vi "SubpanelClosedHandler.vi"(8 "error in (no error)":errorcluster, 9 "UI State":T1=enum."Embedded", 10 "EmbeddedSMO":refnum<class "SMO.UI.Embedded.lvclass">, 11 "SMO.UI.MAUI in":refnum<class "SMO.UI.MAUI.lvclass">) -> (0 "error out":errorcluster, 3 "SMO.UI.MAUI out":refnum<class "SMO.UI.MAUI.lvclass">)   [LabVIEW 2016, in "SMO.UI.MAUI.lvclass"]
uses:
  SMO.UI.MAUI.lvclass
  <vilib>/Levylab/SMO.UI.Embedded/SMO.UI.Embedded.lvclass
  C:/Program Files (x86)/National Instruments/LabVIEW 2016/vi.lib/JKI/JKI SMO/SMO/SMO.lvclass
  <vilib>/Levylab/SMO.UI.Embedded/Typedefs/UI State.ctl
  SMO.UI.MAUI.lvclass/SMO.UI.MAUI.ctl
  <vilib>/JKI/JKI SMO/SMO/SMO.lvclass
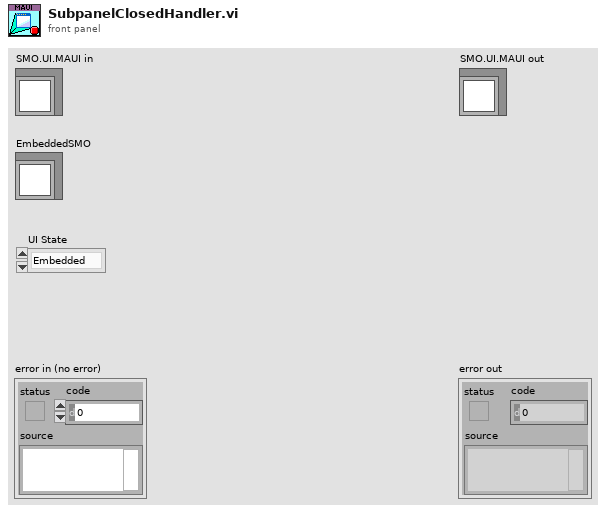
[diagram p1: front panel]
types:
  T1 = typedef "SMO.UI.Embedded.lvclass/UI State.ctl" = enum16{"unknown", "Opened", "Embedded", "Closed"}
  T2 = typedef "SMO.UI.MAUI.lvclass/PanelData.ctl" = cluster{"SubPanel":refnum<vi>, "Ring":refnum<vi>, "Active":i32}
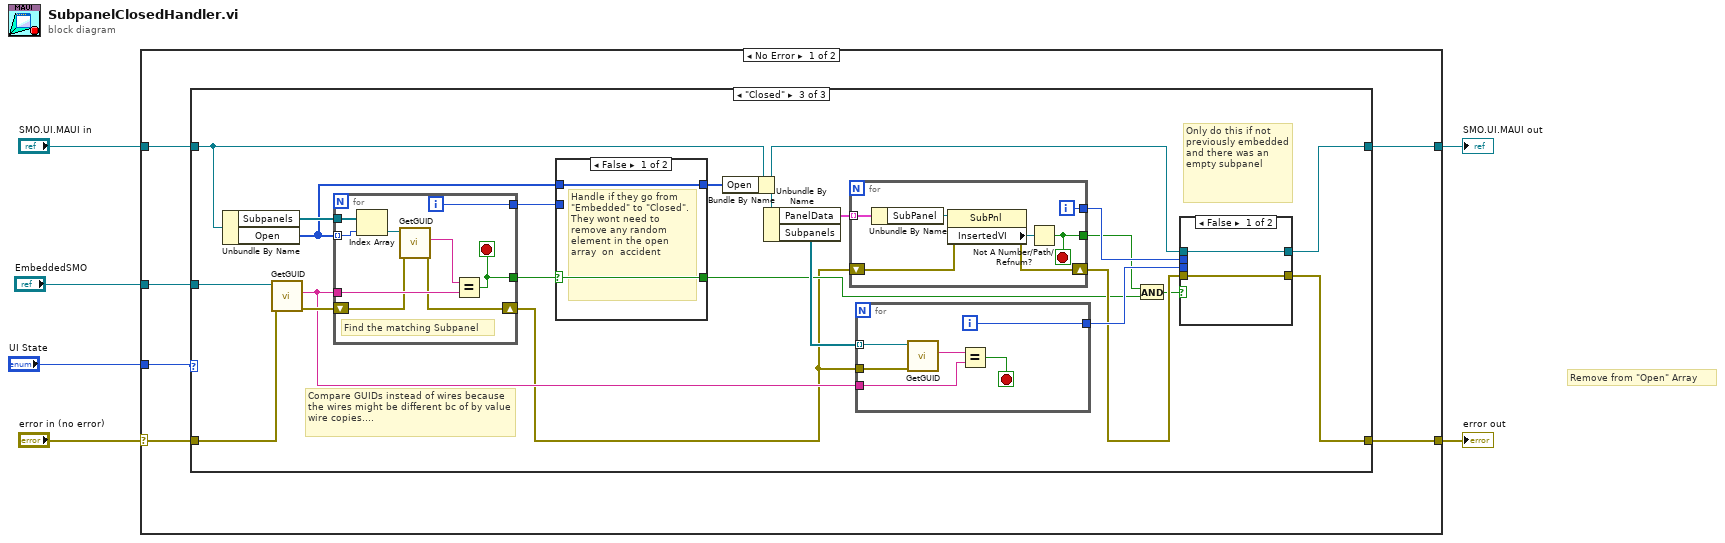
[diagram p0: block diagram]
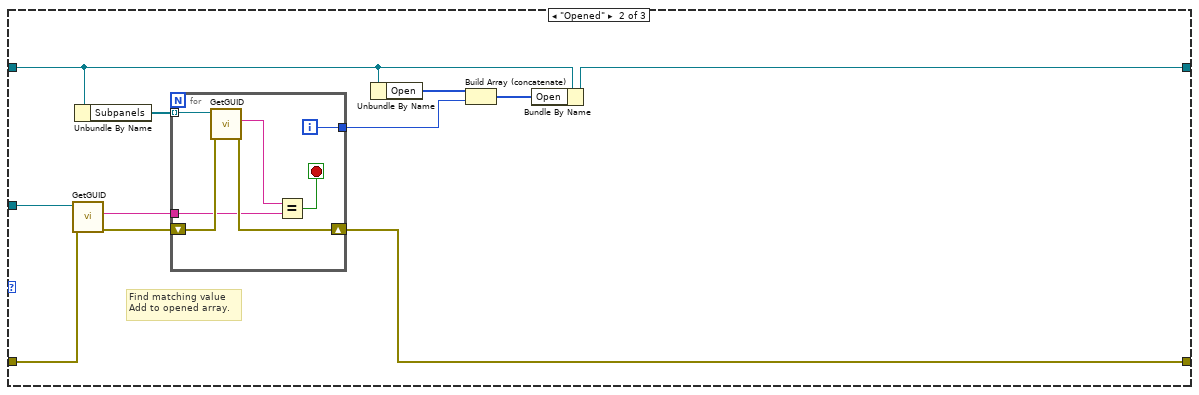
[diagram p3: hidden frame]
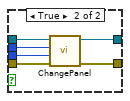
[diagram p4: hidden frame]
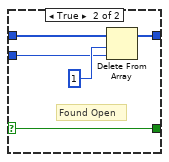
[diagram p5: hidden frame]
diagram:
  # "Remove from \"Open\" Array"
  n1 = case shown="No Error" "error in (no error)" {
    selector: "error in (no error)" -> [w9 w93]
    tunnel: [w8 w93] -> w5
    tunnel: [w11 w92] -> w3
    tunnel: "SMO.UI.MAUI in" -> [w12 w92]
    tunnel: "EmbeddedSMO" -> [w10 _]
    tunnel: "UI State" -> [w7 _]
    frame No Error {
      n2 = case shown="\"Closed\"" w7 {
        tunnel: w12 -> [w14 w19 w52]
        tunnel: [w14 w18 w39] -> w11
        tunnel: w10 -> [_ w24 w45]
        tunnel: w9 -> [w13 w16 w48]
        tunnel: [w13 w15 w37] -> w8
        frame Default {
        }
        frame "Opened" {
          # "Find matching value\nAdd to opened array."
          n3 = call <vilib>:"GetGUID.vi"("error in (no error)"=w16, "SMO"=w24) -> ("error out"=w23:errorcluster, "GUID"=w22:string)  [unwired: 7 in, 1 out]
          n4 = Unbundle By Name(w19) -> ("Subpanels"=w25:refnum<class "SMO.UI.Embedded.lvclass">[])
          n5 = for {
            tunnel: w25 -> [w32] mode=indexing
            shift-right: [w30] -> w15
            shift-left: w23 -> [w31]
            tunnel: w22 -> [w28]
            tunnel: [w26] -> w20
            i -> [w26]
            stop <- w27 stop-if-true
            n6 = call <vilib>:"GetGUID.vi"("error in (no error)"=w31, "SMO"=w32) -> ("error out"=w30:errorcluster, "GUID"=w29:string)  [unwired: 7 in, 1 out]
            n7 = Equal?(x=w29, y=w28) -> (x = y?=w27:bool)
          }
          n8 = Unbundle By Name(w19) -> ("Open"=w21:i32[])
          n9 = Build Array (concatenate)(w21, w20) -> (w17:i32[])
          n10 = Bundle By Name(cluster=w19, "Open"=w17) -> (w18:refnum<class "SMO.UI.MAUI.lvclass">)
        }
        frame "Closed" {
          # "Only do this if not previously embedded and there was an empty subpanel"
          # "Compare GUIDs instead of wires because the wires might be different bc of by value wire copies...."
          n11 = Unbundle By Name(w52) -> ("Subpanels"=w54:refnum<class "SMO.UI.Embedded.lvclass">[], "Open"=w53:i32[])
          n12 = call <vilib>:"GetGUID.vi"("error in (no error)"=w48, "SMO"=w45) -> ("error out"=w49:errorcluster, "GUID"=w43:string)  [unwired: 7 in, 1 out]
          n13 = for {
            tunnel: w54 -> [w91]
            tunnel: w53 -> [w90] mode=indexing
            tunnel: [w87] -> w50
            tunnel: w43 -> [w86]
            shift-right: [w84] -> w33
            shift-left: w49 -> [w85]
            tunnel: [w83] -> w47
            i -> [w87]
            stop <- w83 stop-if-true
            # "Find the matching Subpanel"
            n14 = Index Array(array=w91, index=w90) -> (element=w89:refnum<class "SMO.UI.Embedded.lvclass">)
            n15 = call <vilib>:"GetGUID.vi"("error in (no error)"=w85, "SMO"=w89) -> ("error out"=w84:errorcluster, "GUID"=w88:string)  [unwired: 7 in, 1 out]
            n16 = Equal?(x=w88, y=w86) -> (x = y?=w83:bool)
          }
          n17 = case shown="False" w47 {
            selector: w47 -> [w76 w78]
            tunnel: w53 -> [w77 w82]
            tunnel: [w77 w80] -> w51
            tunnel: w50 -> [_ w79]
            tunnel: [w76 w78] -> w34
            frame False {
              # "Handle if they go from \"Embedded\" to \"Closed\". They wont need to remove any random element in the open array  on  accident"
            }
            frame True {
              # "Found Open"
              n18 = Delete From Array(array=w82, length=1, index=w79) -> (array with subset deleted=w80:i32[])  [unwired: 1 out]
            }
          }
          n19 = Bundle By Name(cluster=w52, "Open"=w51) -> (w40:refnum<class "SMO.UI.MAUI.lvclass">)
          n20 = Unbundle By Name(w40) -> ("PanelData"=w46:T2[], "Subpanels"=w42:refnum<class "SMO.UI.Embedded.lvclass">[])
          n21 = for {
            tunnel: w46 -> [w75] mode=indexing
            tunnel: [w72] -> w36
            tunnel: [w71] -> w44
            shift-right: [w69] -> w38
            shift-left: w33 -> [w70]
            i -> [w71]
            stop <- w72 stop-if-true
            n22 = Unbundle By Name(w75) -> ("SubPanel"=w74:refnum<vi>)
            n23 = property class="SubPnl"(reference=w74, error in=w70) -> (error out=w69:errorcluster, "InsertedVI"=w73:refnum<vi>)  [unwired: 1 out]
            n24 = Not A Number/Path/Refnum?(number/path/refnum=w73) -> (NaN/Path/Refnum?=w72:bool)
          }
          n25 = for {
            tunnel: w43 -> [w66]
            tunnel: w42 -> [w68] mode=indexing
            tunnel: [w64] -> w41
            tunnel: w33 -> [w63]
            i -> [w64]
            stop <- w65 stop-if-true
            n26 = call <vilib>:"GetGUID.vi"("error in (no error)"=w63, "SMO"=w68) -> ("GUID"=w67:string)  [unwired: 7 in, 2 out]
            n27 = Equal?(x=w67, y=w66) -> (x = y?=w65:bool)
          }
          n28 = And(x=w36, y=w34) -> (x .and. y?=w35:bool)
          n29 = case shown="False" w35 {
            tunnel: w44 -> [_ w62]
            tunnel: w41 -> [_ w61]
            tunnel: w40 -> [w56 w60]
            tunnel: [w56 w59] -> w39
            tunnel: w38 -> [w55 w58]
            tunnel: [w55 w57] -> w37
            frame False {
            }
            frame True {
              n30 = call "ChangePanel.vi"("error in (no error)"=w58, "New Active Index"=w61, "Panel Index"=w62, "MAUI in"=w60) -> ("error out"=w57:errorcluster, "MAUI out"=w59:refnum<class "SMO.UI.MAUI.lvclass">)  [unwired: 6 in]
            }
          }
        }
      }
    }
    frame Error {
    }
  }
  "error out" <- w5
  "SMO.UI.MAUI out" <- w3
